vi "数值上升沿.vi"(1 "数值":i16) -> (0 "变化边沿":bool)   [LabVIEW 2014]
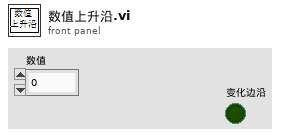
[diagram p1: front panel]
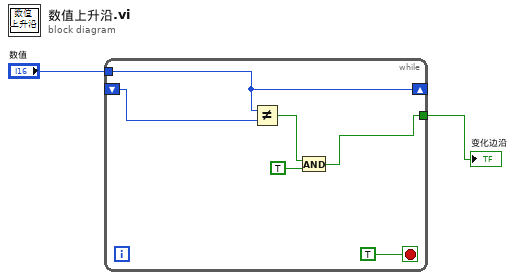
[diagram p0: block diagram]
diagram:
  n1 = while {
    shift-right: [w6] -> _
    shift-left: _ -> [w8]
    tunnel: [w4] -> w2
    tunnel: "数值" -> [w6]
    stop <- TRUE stop-if-true
    n2 = Not Equal?(x=w6, y=w8) -> (x != y?=w5:bool)
    n3 = And(x=w5, y=TRUE) -> (x .and. y?=w4:bool)
  }
  "变化边沿" <- w2
